vi "Destroy My API.vi"(8 "error in (no error)":errorcluster, 11 "My API in":refnum<class "My API.lvclass">) -> (0 "error out":errorcluster)   [LabVIEW 2017, in "My API.lvclass"]
uses:
  My API.lvclass
  My API.lvclass/My API.ctl
  classes/REST Client/REST Client.lvclass
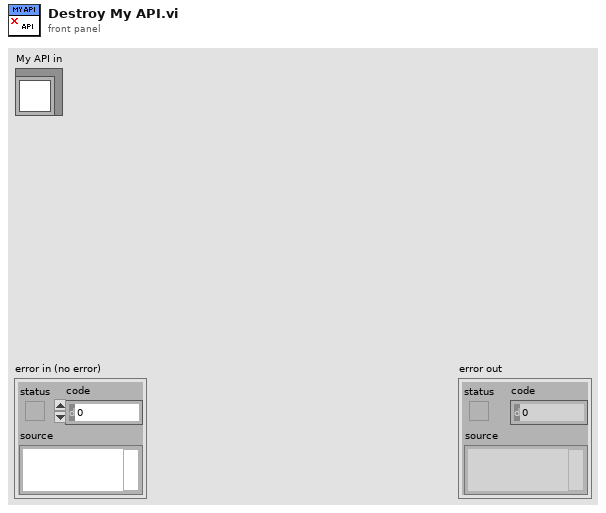
[diagram p1: front panel]
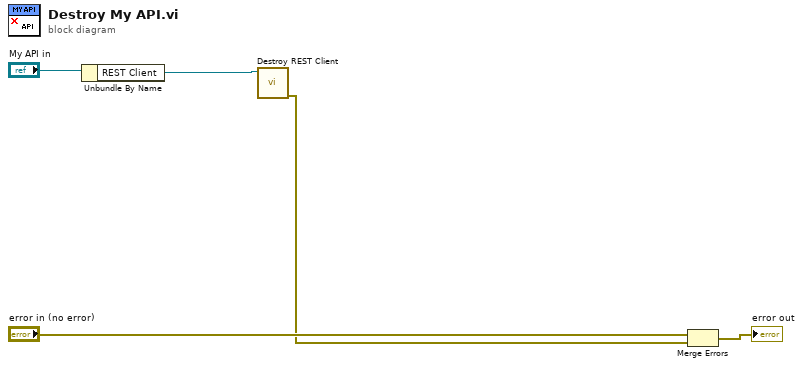
[diagram p0: block diagram]
diagram:
  n1 = Unbundle By Name("My API in") -> ("REST Client"=w2:refnum<class "REST Client.lvclass">)
  n2 = call-dynamic "Destroy REST Client.vi"("REST Client in"=w2) -> ("error out"=w1:errorcluster)  [unwired: 10 in]
  n3 = Merge Errors("error in (no error)", w1) -> (→"error out":errorcluster)
